vi "AttrMap-UnpackMap.vi"(11 "Map":variant) -> (3 "AttrMap":T1)   [LabVIEW 2019, in "lv-apt-json-file.lvlib"]
uses:
  lv-apt-json-file.lvlib
  Def-AttrMap -- Map.ctl
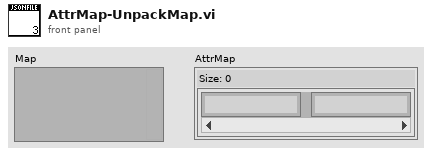
[diagram p1: front panel]
types:
  T1 = typedef "lv-apt-json-file.lvlib/Def-AttrMap -- Map.ctl" = map{string, string}
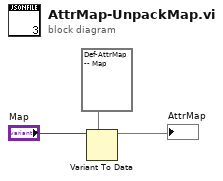
[diagram p0: block diagram]
diagram:
  n1 = Variant To Data(type=T1 {} ("AttrMap"), Variant="Map") -> (data=→"AttrMap":T1)  [unwired: 1 in, 1 out]
